vi "magnet_calibration.vi"() -> ()   [LabVIEW 2016]
uses:
  <vilib>/DAQmx/write.llb/DAQmx Write (Analog DBL 1Chan 1Samp).vi
  <vilib>/DAQmx/create/channels.llb/DAQmx Create Channel (AO-Voltage-Basic).vi
  <vilib>/DAQmx/miscellaneous.llb/DAQmx Fill In Error Info.vi
panel:
  out "error out":errorcluster
  in  "Gaussmeter Name (in)":refnum<visa-resource-name>="Lakeshore_475"
  in  "Time to wait (ms)":dbl=2000.0
  in  "Voltage step (V)":dbl=0.02
  in  "Stop Voltage (V)":dbl=4.0
  in  "Start Voltage (V)":dbl=-4.0
  in  "Error (in)":errorcluster
  in  "DAQ channel (in)":tag="DAQ_6363/ao1"
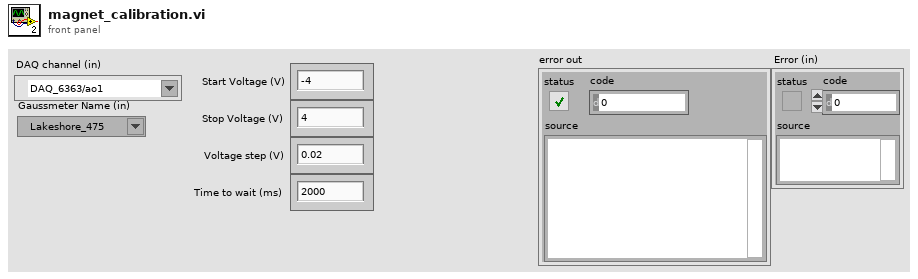
[diagram p1: front panel]
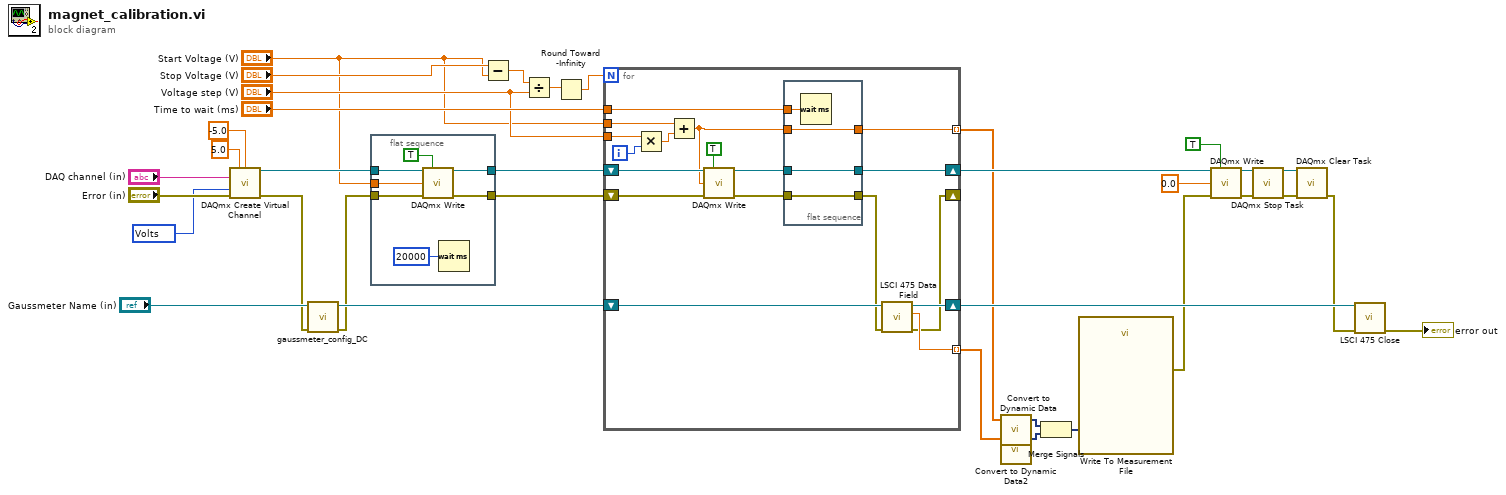
[diagram p0: block diagram]
diagram:
  w31 = 10348 items=["Volts"=10348, "From Custom Scale"=10065] ("units")
  n1 = call-poly <vilib>:"DAQmx Create Virtual Channel.vi"("maximum value"=5.0, "minimum value"=-5.0, "physical channels"="DAQ channel (in)", "units"=w31, "error in"="Error (in)") -> ("task out"=w5:refnum<k21>, "error out"=w25:errorcluster)  [unwired: 9 in]
  n2 = call "gaussmeter_config_DC.vi"("error in (no error)"=w25, "VISA Refnum in"="Gaussmeter Name (in)") -> ("error out"=w4:errorcluster, "VISA Refnum out"=w24:refnum<visa-resource-name>)  [unwired: 8 in]
  n3 = flat-sequence {
    tunnel: w5 -> [w42]
    tunnel: w4 -> [w41]
    tunnel: [w40] -> w3
    tunnel: [w39] -> w2
    tunnel: "Start Voltage (V)" -> [w37]
    frame #0 {
      n4 = call-poly <vilib>:"DAQmx Write.vi"("task/channels in"=w42, "auto start"=TRUE, "data"=w37, "error in"=w41) -> ("task out"=w39:refnum<k21>, "error out"=w40:errorcluster)  [unwired: 9 in, 1 out]
      n5 = Wait (ms)(milliseconds to wait=u32 20000) -> ()  [unwired: 1 out]
    }
  }
  n6 = Subtract(x="Stop Voltage (V)", y="Start Voltage (V)") -> (x-y=w30:dbl)
  n7 = Divide(x=w30, y="Voltage step (V)") -> (x/y=w29:dbl)
  n8 = Round Toward -Infinity(1:w29) -> (0:w28:dbl)
  n9 = for {
    N: w28 -> [_]
    tunnel: "Time to wait (ms)" -> [w60]
    shift-right: [w43] -> w23
    shift-left: w2 -> [w58]
    shift-right: [w54] -> w20
    shift-left: w24 -> [w59]
    tunnel: [w53] -> w8 mode=indexing
    tunnel: [w45] -> w9 mode=indexing
    tunnel: "Start Voltage (V)" -> [w52]
    tunnel: "Voltage step (V)" -> [w51]
    shift-right: [w49] -> _
    shift-left: w3 -> [w50]
    i -> [w57]
    n10 = Multiply(x=w51, y=w57) -> (x*y=w56:dbl)
    n11 = Add(x=w52, y=w56) -> (x+y=w46:dbl)
    n12 = call-poly <vilib>:"DAQmx Write.vi"("task/channels in"=w58, "auto start"=TRUE, "data"=w46, "error in"=w50) -> ("task out"=w44:refnum<k21>, "error out"=w48:errorcluster)  [unwired: 9 in, 1 out]
    n13 = flat-sequence {
      tunnel: w60 -> [w64]
      tunnel: [w63] -> w47
      tunnel: w48 -> [w63]
      tunnel: [w62] -> w45
      tunnel: w46 -> [w62]
      tunnel: [w61] -> w43
      tunnel: w44 -> [w61]
      frame #0 {
        n14 = Wait (ms)(milliseconds to wait=w64) -> ()  [unwired: 1 out]
      }
    }
    n15 = call <instrlib>:"LSCI 475 Data Field.vi"("error in (no error)"=w47, "VISA session"=w59) -> ("error out"=w49:errorcluster, "Field Reading"=w53:dbl, "dup VISA session"=w54:refnum<visa-resource-name>)  [unwired: 7 in]
  }
  n16 = call "Convert to Dynamic Data"("Array"=w9) -> ("Dynamic Data Type"=w12:dynamicdata)  [unwired: 3 in]
  n17 = call "Convert to Dynamic Data2"("Array"=w8) -> ("Dynamic Data Type"=w10:dynamicdata)  [unwired: 3 in]
  n18 = Merge Signals(w12, w10) -> (w11:dynamicdata)
  n19 = call "Write To Measurement File"("Signals"=w11) -> ("error out"=w13:errorcluster)  [unwired: 16 in, 2 out]
  n20 = call-poly <vilib>:"DAQmx Write.vi"("task/channels in"=w23, "auto start"=TRUE, "data"=0.0, "error in"=w13) -> ("task out"=w16:refnum<k21>, "error out"=w15:errorcluster)  [unwired: 9 in, 1 out]
  n21 = call <vilib>:"DAQmx Stop Task.vi"("task/channels in"=w16, "error in"=w15) -> ("task out"=w18:refnum<k21>, "error out"=w17:errorcluster)  [unwired: 12 in]
  n22 = call <vilib>:"DAQmx Clear Task.vi"("task in"=w18, "error in"=w17) -> ("error out"=w14:errorcluster)  [unwired: 13 in]
  n23 = call <instrlib>:"LSCI 475 Close.vi"("VISA session"=w20, "error in (no error)"=w14) -> ("error out"=→"error out":errorcluster)  [unwired: 13 in]
